vi "update.vi"(8 "error in (no error)":errorcluster, 10 "adapter executability":T1={"instrument"=TRUE, "trajectory"=TRUE, "scanHead"=TRUE, "DAQ"=TRUE, "imageAssembler"=TRUE, "dataCollection"=TRUE, "display"=TRUE, "analyser"=TRUE, "stimulator"=TRUE}, 11 "ScanModeMG091111IntrinsicImaging in":refnum<class "ImagingModeMG091111IntrinsicImaging.lvclass">) -> (0 "error out":errorcluster, 3 "ScanModeMG091111IntrinsicImaging out":refnum<class "ImagingModeMG091111IntrinsicImaging.lvclass">)   [LabVIEW 2010, in "ImagingModeMG091111IntrinsicImaging.lvclass"]
uses:
  ImagingModeMG091111IntrinsicImaging.lvclass
  ImagingModeDL090923Scaffold/ImagingModeDL090923Scaffold/adapter_executability_cluster.ctl
  ImagingModeDL091001Scaffold/ImagingModeDL091001Scaffold/ImagingModeDL091001Scaffold.lvclass
  DAQ/GenericDAQ/GenericDAQ/GenericDAQ.lvclass
  ImageAssembler/GenericImageAssembler/GenericImageAssembler/GenericImageAssembler.lvclass
  DataCollection/GenericDataCollection/GenericDataCollection/GenericDataCollection.lvclass
  ImagingModeDL090923Scaffold/ImagingModeDL090923Scaffold/ImagingModeDL090923Scaffold.lvclass
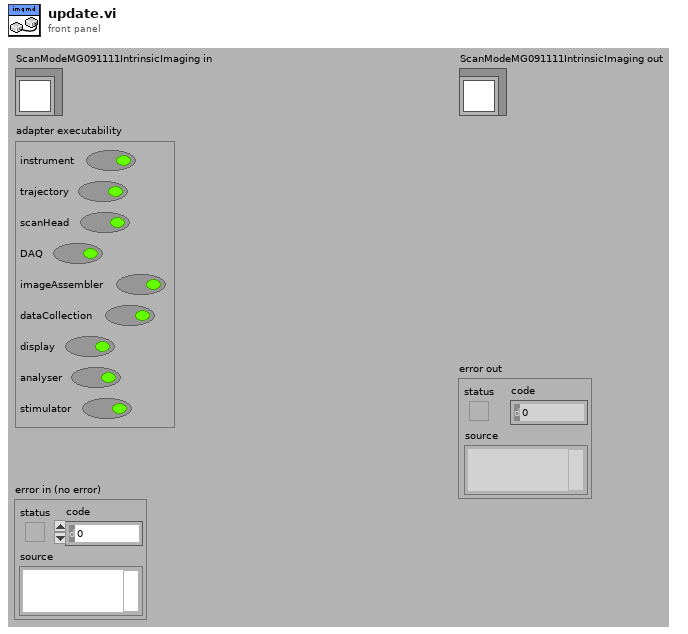
[diagram p1: front panel]
types:
  T1 = typedef "ImagingModeDL090923Scaffold.lvclass/adapter_executability_cluster.ctl" = cluster{"instrument":bool, "trajectory":bool, "scanHead":bool, "DAQ":bool, "imageAssembler":bool, "dataCollection":bool, "display":bool, "analyser":bool, "stimulator":bool}
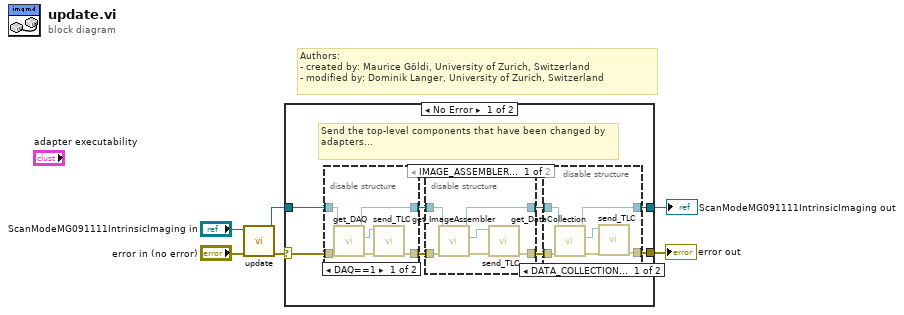
[diagram p0: block diagram]
diagram:
  # "Authors: \n- created by: Maurice Göldi, University of Zurich, Switzerland\n- modified by: Dominik Langer, University of Zurich, Switzerland"
  n1 = call-parent "update.vi"("error in (no error)"="error in (no error)", "ScanModeDL090923Scaffold in"="ScanModeMG091111IntrinsicImaging in") -> ("error out"=w1:errorcluster, "ScanModeDL090923Scaffold out"=w3:refnum<class "ImagingModeMG091111IntrinsicImaging.lvclass">)  [unwired: 8 in]
  n2 = case shown="No Error" w1 {
    selector: w1 -> [w14 w39]
    tunnel: [w12 w39] -> w4
    tunnel: w3 -> [w13 w40]
    tunnel: [w11 w40] -> w2
    frame No Error {
      # "Send the top-level components that have been changed by adapters..."
      n3 = disable-structure shown="DAQ==1" {
        disable-tunnel: [w36 w37] -> w7
        disable-tunnel: w13 -> [w35 w37]
        disable-tunnel: w14 -> [w34 w38]
        disable-tunnel: [w32 w38] -> w10
        frame condition #0 {
          n4 = call-dynamic "get_DAQ.vi"("error in (no error)"=w34, "ScanModeDL090923Scaffold in"=w35) -> ("error out"=w33:errorcluster, "DAQ"=w31:refnum<class "GenericDAQ.lvclass">, "ScanModeDL090923Scaffold out"=w36:refnum<class "ImagingModeMG091111IntrinsicImaging.lvclass">)  [unwired: 4 in, 3 out]
          n5 = call-dynamic "send_TLC.vi"("error in (no error)"=w33, "GenericToplevelComponent in"=w31) -> ("error out"=w32:errorcluster)  [unwired: 8 in, 1 out]
        }
        frame condition #1 (active) {
        }
      }
      n6 = disable-structure shown="IMAGE_ASSEMBLER==1" {
        disable-tunnel: w10 -> [w26 w30]
        disable-tunnel: [w25 w30] -> w9
        disable-tunnel: [w24 w29] -> w8
        disable-tunnel: w7 -> [w23 w29]
        frame condition #0 {
          n7 = call-dynamic "get_ImageAssembler.vi"("error in (no error)"=w26, "ScanModeDL090923Scaffold in"=w23) -> ("error out"=w28:errorcluster, "ImageAssembler"=w27:refnum<class "GenericImageAssembler.lvclass">, "ScanModeDL090923Scaffold out"=w24:refnum<class "ImagingModeMG091111IntrinsicImaging.lvclass">)  [unwired: 4 in, 3 out]
          n8 = call-dynamic "send_TLC.vi"("error in (no error)"=w28, "GenericToplevelComponent in"=w27) -> ("error out"=w25:errorcluster)  [unwired: 8 in, 1 out]
        }
        frame condition #1 (active) {
        }
      }
      n9 = disable-structure shown="DATA_COLLECTION==1" {
        disable-tunnel: [w18 w22] -> w12
        disable-tunnel: [w17 w21] -> w11
        disable-tunnel: w9 -> [w16 w22]
        disable-tunnel: w8 -> [w15 w21]
        frame condition #0 {
          n10 = call-dynamic "get_DataCollection.vi"("error in (no error)"=w16, "ScanModeDL090923Scaffold in"=w15) -> ("error out"=w20:errorcluster, "DataCollection"=w19:refnum<class "GenericDataCollection.lvclass">, "ScanModeDL090923Scaffold out"=w17:refnum<class "ImagingModeMG091111IntrinsicImaging.lvclass">)  [unwired: 4 in, 3 out]
          n11 = call-dynamic "send_TLC.vi"("error in (no error)"=w20, "GenericToplevelComponent in"=w19) -> ("error out"=w18:errorcluster)  [unwired: 8 in, 1 out]
        }
        frame condition #1 (active) {
        }
      }
    }
    frame Error {
    }
  }
  "error out" <- w4
  "ScanModeMG091111IntrinsicImaging out" <- w2
